vi "Write Channel Units.vi"(8 "error in (no error)":errorcluster, 10 "Channel Setup":T1, 11 "HK Item in":refnum<class "HK Item.lvclass">) -> (0 "error out":errorcluster, 3 "HK Item out":refnum<class "HK Item.lvclass">)   [LabVIEW 2024, in "HK Item.lvclass"]
uses:
  HK Item.lvclass
  HK Channel Units and Setup.ctl
  HK Channel enum Data Type.ctl
  HK Item.lvclass/HK Item.ctl
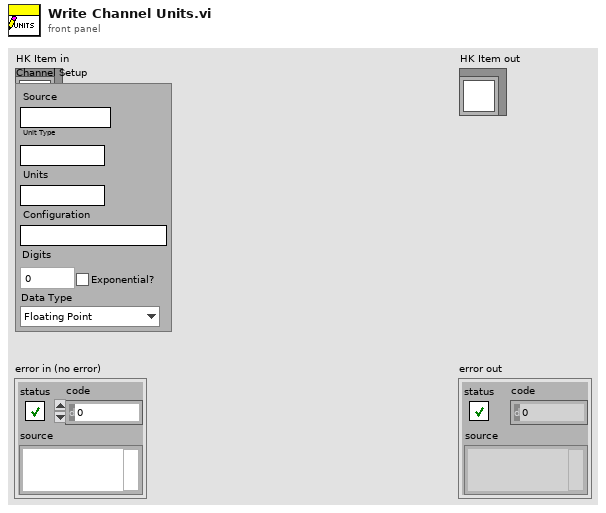
[diagram p1: front panel]
types:
  T1 = typedef "HK Item.lvclass/HK Channel Units and Setup.ctl" = cluster{"Unit Type":string, "Units":string, "Configuration":string, "Digits":i32, "Data Type":T2, "Exponential?":bool, "Source":string}
  T2 = typedef "HK Item.lvclass/HK Channel enum Data Type.ctl" = enum16{"Floating Point", "Integer", "Enum", "String", "Waveform", "File"}
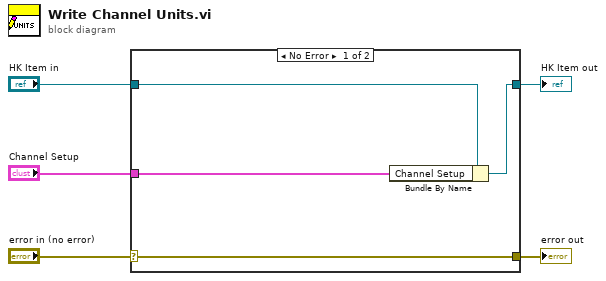
[diagram p0: block diagram]
diagram:
  n1 = case shown="No Error" "error in (no error)" {
    selector: "error in (no error)" -> [w9 w10]
    tunnel: [w9 w10] -> w4
    tunnel: [w7 w11] -> w2
    tunnel: "HK Item in" -> [w8 w11]
    tunnel: "Channel Setup" -> [w6 _]
    frame No Error {
      n2 = Bundle By Name(cluster=w8, "Channel Setup"=w6) -> (w7:refnum<class "HK Item.lvclass">)
    }
    frame Error {
    }
  }
  "error out" <- w4
  "HK Item out" <- w2
